vi "svfa_Convert to One-Sided Power Spectrum.vi"(0 "two-sided power spectrum":dbl[](array[numeric]) format="%.2f") -> (1 "one-sided power spectrum":dbl[](array[numeric]) format="%.2f", 2 "block size":dbl format="%.2f")   [LabVIEW 2017]
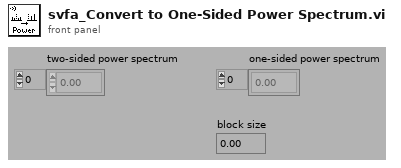
[diagram p1: front panel]
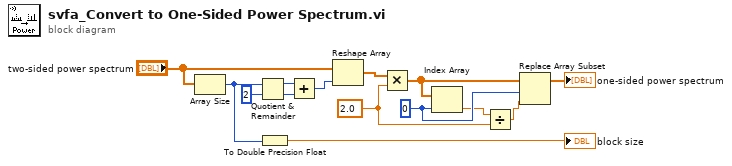
[diagram p0: block diagram]
diagram:
  w3 = 2.0
  w13 = 0
  n1 = Array Size(array="two-sided power spectrum") -> (size(s)=w7:i32)
  n2 = Quotient & Remainder(x=w7, y=2) -> (x-y*floor(x/y)=w11:i32, floor(x/y)=w10:i32)
  n3 = To Double Precision Float(number=w7) -> (double precision float=→"block size":dbl)
  n4 = Add(x=w11, y=w10) -> (x+y=w9:i32)
  n5 = Reshape Array("two-sided power spectrum", w9) -> (w5:dbl[])
  n6 = Multiply(x=w5, y=w3) -> (x*y=w4:dbl[])
  n7 = Index Array(array=w4, index=w13) -> (element=w2:dbl)
  n8 = Divide(x=w2, y=w3) -> (x/y=w1:dbl)
  n9 = Replace Array Subset(array=w4, new element=w1, index=w13) -> (→"one-sided power spectrum":dbl[])
